vi "test Read All Commands.vi"() -> (0 "error out":errorcluster, 2 "pass?":bool)   [LabVIEW 2019, in "RESP3 Tests.lvlib"]
uses:
  RESP3 Tests.lvlib
  RESP3/types/RESP3 Type.ctl
  RESP3/RESP3 Parser/RESP3 Parser.lvclass
  RESP3/types/RESP3 data type attribute.vi
  RESP3/RESP3.lvlib
panel:
  out "parse time (ms)":dbl
  out "COMMANDs":T1(array[cluster])
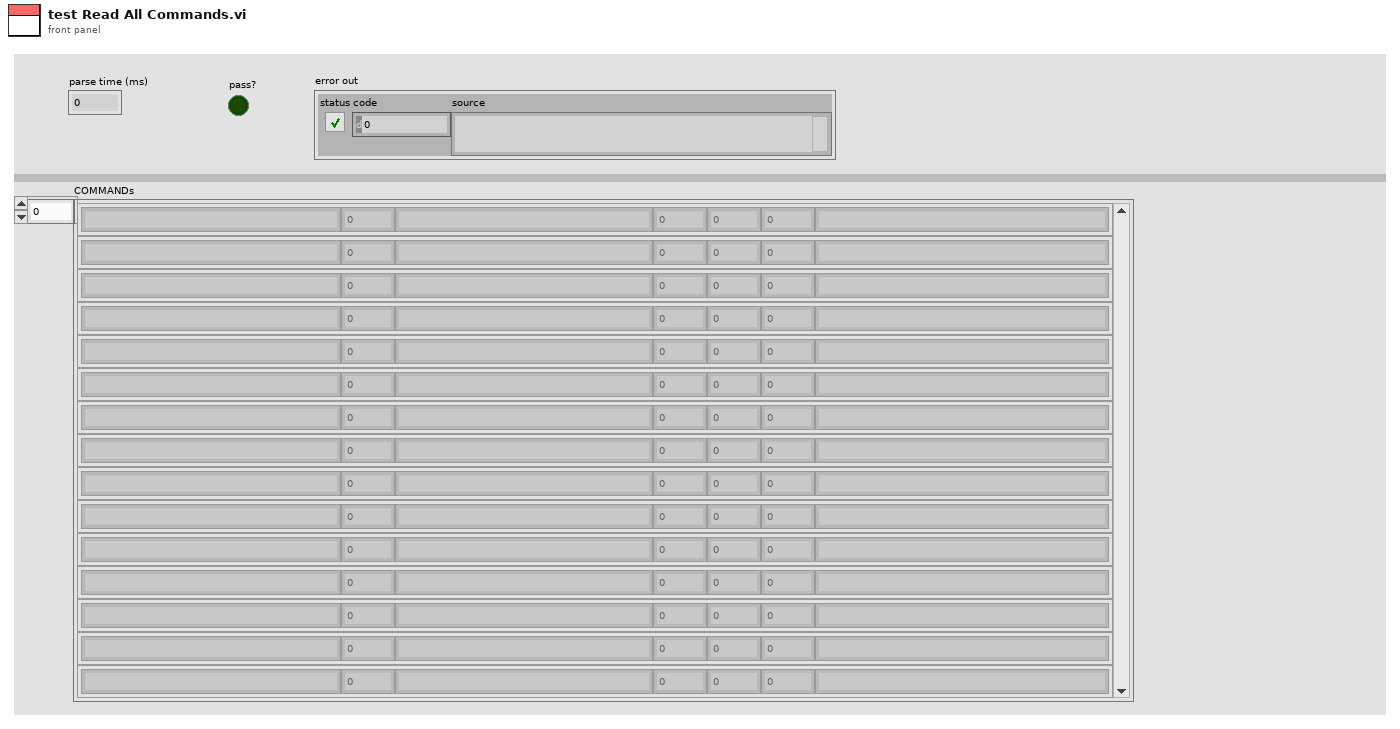
[diagram p1: front panel]
types:
  T1 = cluster{string, i64, "trimmed string":string, i64, i64, i64, "trimmed string":string}[]
  T2 = typedef "RESP3.lvlib/RESP3 Type.ctl" = enum8{"<0x00>", "<0x01>", "<0x02>", "<0x03>", "<0x04>", "<0x05>", "<0x06>", "<0x07>", "<0x08>", "<0x09>", "<0x0A>", "<0x0B>", "<0x0C>", "<0x0D>", "<0x0E>", "<0x0F>", "<0x10>", "<0x11>", "<0x12>", "<0x13>", "<0x14>", "<0x15>", "<0x16>", "<0x17>", "<0x18>", "<0x19>", "<0x1A>", "<0x1B>", "<0x1C>", "<0x1D>", "<0x1E>", "<0x1F>", "\" \"", "BLOB ERROR", "\"\"\"", "BOOLEAN", "BLOB", "MAP", "\"&\"", "\"'\"", "BIG NUMBER", "\")\"", "ARRAY", "STRING", "DOUBLE", "ERROR", "END", "\"/\"", "\"0\"", "\"1\"", "\"2\"", "\"3\"", "\"4\"", "\"5\"", "\"6\"", "\"7\"", "\"8\"", "\"9\"", "INTEGER", "STREAM", "\"<\"", "VERBATIM STRING", "PUSH", "\"?\"", "\"@\"", "\"A\"", "\"B\"", "\"C\"", "\"D\"", "\"E\"", "\"F\"", "\"G\"", "\"H\"", "\"I\"", "\"J\"", "\"K\"", "\"L\"", "\"M\"", "\"N\"", "\"O\"", "\"P\"", "\"Q\"", "\"R\"", "\"S\"", "\"T\"", "\"U\"", "\"V\"", "\"W\"", "\"X\"", "\"Y\"", "\"Z\"", "\"[\"", "\"\\\"", "\"]\"", "\"^\"", "NULL", "\"`\"", "\"a\"", "\"b\"", "\"c\"", "\"d\"", "\"e\"", "\"f\"", "\"g\"", "\"h\"", "\"i\"", "\"j\"", "\"k\"", "\"l\"", "\"m\"", "\"n\"", "\"o\"", "\"p\"", "\"q\"", "\"r\"", "\"s\"", "\"t\"", "\"u\"", "\"v\"", "\"w\"", "\"x\"", "\"y\"", "\"z\"", "\"{\"", "ATTRIBUTES", "\"}\"", "SET", "<0x7F>", "<0x80>", "<0x81>", "<0x82>", "<0x83>", "<0x84>", "<0x85>", "<0x86>", "<0x87>", "<0x88>", "<0x89>", "<0x8A>", "<0x8B>", "<0x8C>", "<0x8D>", "<0x8E>", "<0x8F>", "<0x90>", "<0x91>", "<0x92>", "<0x93>", "<0x94>", "<0x95>", "<0x96>", "<0x97>", "<0x98>", "<0x99>", "<0x9A>", "<0x9B>", "<0x9C>", "<0x9D>", "<0x9E>", "<0x9F>", "<0xA0>", "<0xA1>", "<0xA2>", "<0xA3>", "<0xA4>", "<0xA5>", "<0xA6>", "<0xA7>", "<0xA8>", "<0xA9>", "<0xAA>", "<0xAB>", "<0xAC>", "<0xAD>", "<0xAE>", "<0xAF>", "<0xB0>", "<0xB1>", "<0xB2>", "<0xB3>", "<0xB4>", "<0xB5>", "<0xB6>", "<0xB7>", "<0xB8>", "<0xB9>", "<0xBA>", "<0xBB>", "<0xBC>", "<0xBD>", "<0xBE>", "<0xBF>", "<0xC0>", "<0xC1>", "<0xC2>", "<0xC3>", "<0xC4>", "<0xC5>", "<0xC6>", "<0xC7>", "<0xC8>", "<0xC9>", "<0xCA>", "<0xCB>", "<0xCC>", "<0xCD>", "<0xCE>", "<0xCF>", "<0xD0>", "<0xD1>", "<0xD2>", "<0xD3>", "<0xD4>", "<0xD5>", "<0xD6>", "<0xD7>", "<0xD8>", "<0xD9>", "<0xDA>", "<0xDB>", "<0xDC>", "<0xDD>", "<0xDE>", "<0xDF>", "<0xE0>", "<0xE1>", "<0xE2>", "<0xE3>", "<0xE4>", "<0xE5>", "<0xE6>", "<0xE7>", "<0xE8>", "<0xE9>", "<0xEA>", "<0xEB>", "<0xEC>", "<0xED>", "<0xEE>", "<0xEF>", "<0xF0>", "<0xF1>", "<0xF2>", "<0xF3>", "<0xF4>", "<0xF5>", "<0xF6>", "<0xF7>", "<0xF8>", "<0xF9>", "<0xFA>", "<0xFB>", "<0xFC>", "<0xFD>", "<0xFE>"}
  T3 = cluster{string, i64, "trimmed string":string, i64, i64, i64, "trimmed string":string}
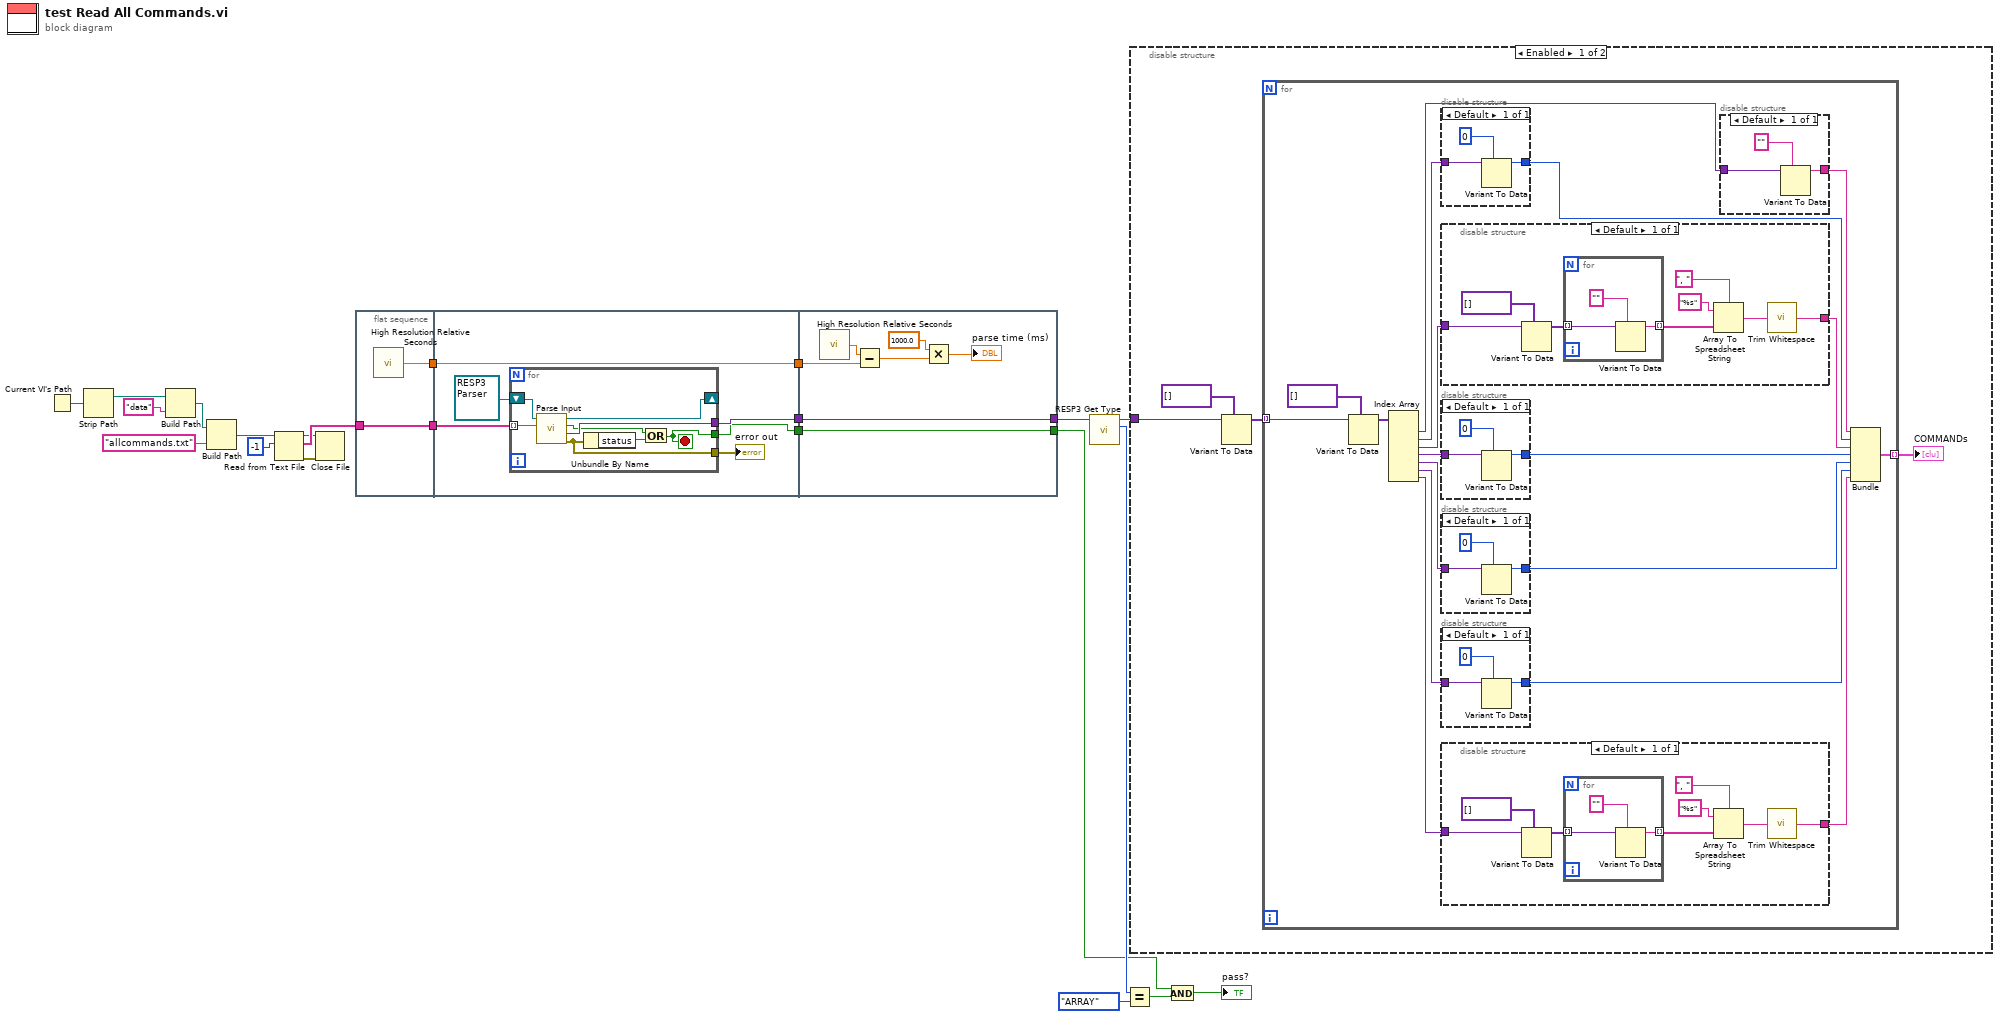
[diagram p0: block diagram]
diagram:
  n1 = Current VI's Path() -> (path=w19:path)
  n2 = Strip Path(path=w19) -> (stripped path=w18:path)  [unwired: 1 out]
  n3 = Build Path(base path=w18, name or relative path="data") -> (appended path=w16:path)
  n4 = Build Path(base path=w16, name or relative path="allcommands.txt") -> (appended path=w14:path)
  n5 = Read from Text File(file (use dialog)=w14, count=-1) -> (refnum out=w11:refnum<file>, text=w12:string[], error out=w10:errorcluster)  [unwired: 2 in, 1 out]
  n6 = Close File(refnum=w11, error in=w10) -> ()  [unwired: 2 out]
  n7 = flat-sequence {
    tunnel: w12 -> [w24]
    tunnel: [w24] -> w3
    tunnel: [w23] -> w2
    tunnel: [w29] -> w5
    tunnel: [w26] -> w4
    tunnel: w3 -> [w28]
    tunnel: w2 -> [w25]
    tunnel: [w25] -> w1
    tunnel: [w44] -> w6
    tunnel: [w45] -> w22
    tunnel: w5 -> [w45]
    tunnel: w4 -> [w44]
    tunnel: w1 -> [w42]
    frame #0 {
      n8 = call <vilib>:"High Resolution Relative Seconds.vi"() -> ("relative seconds"=w23:dbl)
    }
    frame #1 {
      n9 = for {
        shift-right: [w37] -> _
        shift-left: refnum<class "RESP3 Parser.lvclass"> refnum ("RESP3.lvlib:RESP3 Parser.lvclass") -> [w38]
        tunnel: [w36] -> w29
        tunnel: [w34] -> w26
        tunnel: [w32] -> w27
        tunnel: w28 -> [w31] mode=indexing
        stop <- w34 stop-if-true
        n10 = call-dynamic "Parse Input.vi"("input line"=w31, "RESP3 Parser in"=w38) -> ("error out"=w32:errorcluster, "RESP3 Value"=w36:variant, "finished?"=w35:bool, "RESP3 Parser out"=w37:refnum<class "RESP3 Parser.lvclass">)  [unwired: 5 in, 1 out]
        n11 = Unbundle By Name(w32) -> ("status"=w33:bool)
        n12 = Or(x=w35, y=w33) -> (x .or. y?=w34:bool)
      }
      "error out" <- w27
    }
    frame #2 {
      n13 = call <vilib>:"High Resolution Relative Seconds.vi"() -> ("relative seconds"=w43:dbl)
      n14 = Subtract(x=w43, y=w42) -> (x-y=w41:dbl)
      n15 = Multiply(x=1000.0, y=w41) -> (x*y=→"parse time (ms)":dbl)
    }
  }
  n16 = call "RESP3 Get Type.vi"("RESP3 Value in"=w22) -> ("RESP3 Type"=w21:T2, "RESP3 Value out"=w8:variant)  [unwired: 7 in, 2 out]
  n17 = Equal?(x=w21, y=RESP3_Type."ARRAY") -> (x = y?=w9:bool)
  n18 = disable-structure shown="Enabled" {
    disable-tunnel: w8 -> [w48 _]
    frame Enabled {
      n19 = Variant To Data(type=variant[] [], Variant=w48) -> (data=w47:variant[])  [unwired: 1 in, 1 out]
      n20 = for {
        tunnel: w47 -> [w66] mode=indexing
        tunnel: [w50] -> w46 mode=indexing
        n21 = Variant To Data(type=variant[] [], Variant=w66) -> (data=w64:variant[])  [unwired: 1 in, 1 out]
        n22 = Index Array(array=w64) -> (element #1=w65:variant, element #2=w63:variant, element #3=w62:variant, element #4=w61:variant, element #5=w60:variant, element #6=w59:variant, element #7=w58:variant)  [unwired: 7 in]
        n23 = disable-structure shown="Default" {
          disable-tunnel: w63 -> [w78]
          disable-tunnel: [w77] -> w56
          frame Enabled {
            n24 = Variant To Data(type=i64 0, Variant=w78) -> (data=w77:i64)  [unwired: 1 in, 1 out]
          }
        }
        n25 = disable-structure shown="Default" {
          disable-tunnel: w62 -> [w100]
          disable-tunnel: [w94] -> w55
          frame Enabled {
            n26 = Variant To Data(type=variant[] [], Variant=w100) -> (data=w99:variant[])  [unwired: 1 in, 1 out]
            n27 = for {
              tunnel: w99 -> [w103] mode=indexing
              tunnel: [w102] -> w96 mode=indexing
              n28 = Variant To Data(type="", Variant=w103) -> (data=w102:string)  [unwired: 1 in, 1 out]
            }
            n29 = Array To Spreadsheet String(delimiter (Tab)=", ", array=w96, 3:"%s" ("format string")) -> (spreadsheet string=w95:string)
            n30 = call <vilib>:"Trim Whitespace.vi"("string"=w95) -> ("trimmed string"=w94:string)  [unwired: 1 in]
          }
        }
        n31 = disable-structure shown="Default" {
          disable-tunnel: w61 -> [w75]
          disable-tunnel: [w74] -> w54
          frame Enabled {
            n32 = Variant To Data(type=i64 0, Variant=w75) -> (data=w74:i64)  [unwired: 1 in, 1 out]
          }
        }
        n33 = disable-structure shown="Default" {
          disable-tunnel: w60 -> [w72]
          disable-tunnel: [w71] -> w53
          frame Enabled {
            n34 = Variant To Data(type=i64 0, Variant=w72) -> (data=w71:i64)  [unwired: 1 in, 1 out]
          }
        }
        n35 = disable-structure shown="Default" {
          disable-tunnel: w59 -> [w69]
          disable-tunnel: [w68] -> w52
          frame Enabled {
            n36 = Variant To Data(type=i64 0, Variant=w69) -> (data=w68:i64)  [unwired: 1 in, 1 out]
          }
        }
        n37 = disable-structure shown="Default" {
          disable-tunnel: w58 -> [w89]
          disable-tunnel: [w83] -> w51
          frame Enabled {
            n38 = Variant To Data(type=variant[] [], Variant=w89) -> (data=w88:variant[])  [unwired: 1 in, 1 out]
            n39 = for {
              tunnel: w88 -> [w92] mode=indexing
              tunnel: [w91] -> w85 mode=indexing
              n40 = Variant To Data(type="", Variant=w92) -> (data=w91:string)  [unwired: 1 in, 1 out]
            }
            n41 = Array To Spreadsheet String(delimiter (Tab)=", ", array=w85, 3:"%s" ("format string")) -> (spreadsheet string=w84:string)
            n42 = call <vilib>:"Trim Whitespace.vi"("string"=w84) -> ("trimmed string"=w83:string)  [unwired: 1 in]
          }
        }
        n43 = disable-structure shown="Default" {
          disable-tunnel: w65 -> [w81]
          disable-tunnel: [w80] -> w57
          frame Enabled {
            n44 = Variant To Data(type="", Variant=w81) -> (data=w80:string)  [unwired: 1 in, 1 out]
          }
        }
        n45 = Bundle(w57, w56, "trimmed string"=w55, w54, w53, w52, "trimmed string"=w51) -> (w50:T3)  [unwired: 1 in]
      }
      "COMMANDs" <- w46
    }
    frame Disabled {
    }
  }
  n46 = Compound Arithmetic op=AND(w6, w9) -> (→"pass?":bool)
